vi "test data transfer rate.vi"() -> ()   [LabVIEW 2017]
panel:
  in  "File Path Control":path
  out "Temperature":string
  out "RPMs":string
  out "ECU COM Port Out":refnum<visa-resource-name>
  in  "ECU COM Port":refnum<visa-resource-name>
  out "Error Out":errorcluster
  in  "Error In":errorcluster
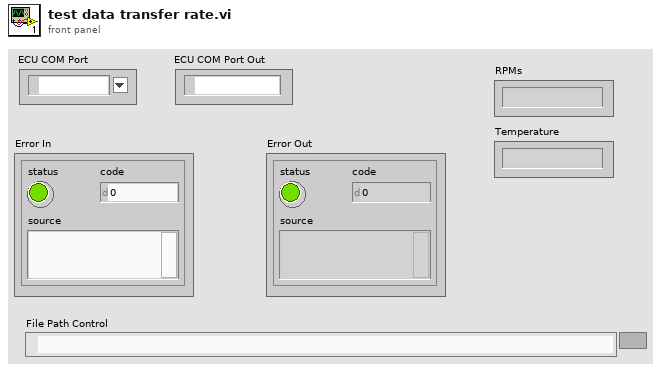
[diagram p1: front panel]
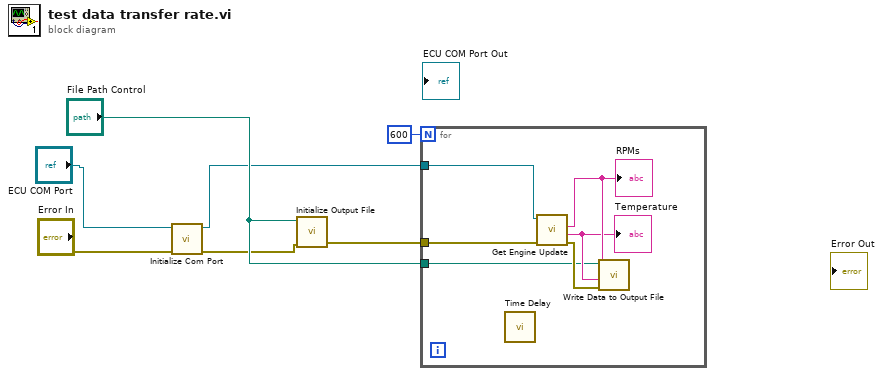
[diagram p0: block diagram]
diagram:
  n1 = call "Initialize Com Port.vi"("Error In"="Error In", "ECU COM Port"="ECU COM Port") -> ("Error Out"=w3:errorcluster, "ECU COM Port Out"=w1:refnum<visa-resource-name>)  [unwired: 8 in]
  n2 = call "Initialize Output File.vi"("error in (no error)"=w3, "File Path Control"="File Path Control") -> ("error out"=w6:errorcluster)  [unwired: 9 in]
  n3 = for {
    N: 600 -> [_]
    tunnel: w6 -> [w13]
    tunnel: w1 -> [w12]
    tunnel: "File Path Control" -> [w8]
    n4 = call "Time Delay"() -> ()  [unwired: 11 in, 1 out]
    n5 = call "Get Engine Update.vi"("Error In"=w13, "ECU COM Port"=w12) -> ("Error Out"=w9:errorcluster, "Temperature"=w10:string, "RPMs"=w11:string)  [unwired: 6 in, 1 out]
    "RPMs" <- w11
    "Temperature" <- w10
    n6 = call "Write Data to Output File.vi"("Error In"=w9, "Temperature"=w10, "RPM"=w11, "File Path Control"=w8) -> ()  [unwired: 7 in, 1 out]
  }
